vi "Volt Data with Time Data.vi"(6 "Use Record Time":bool, 8 "Record Time (s)":dbl=10.0, 9 "Voltage":waveform(dbl)[](array[waveform]), 10 "t_start in":dbl, 11 "dt":dbl) -> (0 "Recording":bool, 1 "timeout":i32, 2 "t_start out":dbl, 3 "Data with Time":dbl[][](array[numeric]))   [LabVIEW 2021]
doc: "This VI helps to create time array and merge it with Voltage Data."
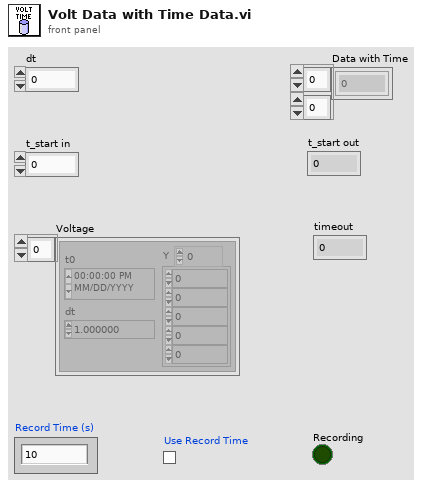
[diagram p1: front panel]
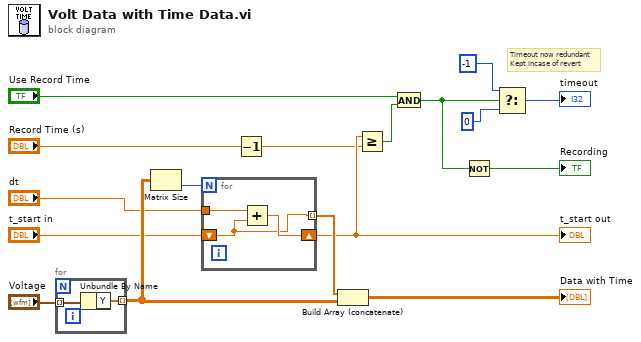
[diagram p0: block diagram]
diagram:
  # "Timeout now redundant\nKept incase of revert"
  n1 = for {
    tunnel: "Voltage" -> [w19] mode=indexing
    tunnel: [w18] -> w17 mode=indexing
    n2 = Unbundle By Name(w19) -> ("Y"=w18:dbl[])
  }
  n3 = Matrix Size(0:w17) -> (2:w16:i32)  [unwired: 1 out]
  n4 = for {
    N: w16 -> [_]
    tunnel: "dt" -> [w21]
    tunnel: [w20] -> w14 mode=indexing
    shift-right: [w22] -> w3
    shift-left: "t_start in" -> [w20]
    n5 = Add(x=w21, y=w20) -> (x+y=w22:dbl)
  }
  "t_start out" <- w3
  n6 = Decrement(x="Record Time (s)") -> (x-1=w1:dbl)
  n7 = Build Array (concatenate)(w14, w17) -> (→"Data with Time":dbl[][])
  n8 = Greater Or Equal?(x=w3, y=w1) -> (x >= y?=w6:bool)
  n9 = And(x="Use Record Time", y=w6) -> (x .and. y?=w5:bool)
  n10 = Not(x=w5) -> (.not. x?=→"Recording":bool)
  n11 = Select(t=-1, s=w5, f=0) -> (s? t:f=→"timeout":i32)
